vi "WritemmWavePosition.vi"(8 "error in (no error)":errorcluster, 9 "Axis Position, eng.":dbl, 10 "mmWave Axis Name":string, 11 "UI MotionStatus in":refnum<class "UI MotionStatus.lvclass">) -> (0 "error out":errorcluster, 3 "UI MotionStatus out":refnum<class "UI MotionStatus.lvclass">)   [LabVIEW 2019, in "UI MotionStatus.lvclass"]
doc: "Use mmWave axis name to find numeric indicator refnum.\nwrite value."
uses:
  UI MotionStatus.lvclass
  UI MotionStatus.lvclass/UI MotionStatus.ctl
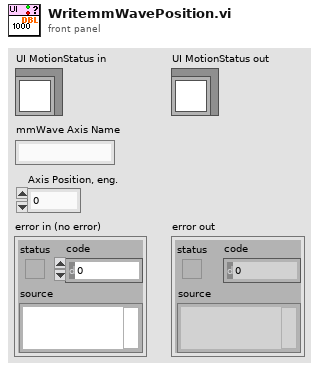
[diagram p1: front panel]
types:
  T1 = typedef "PositonIndicatorsCtrlRefs.ctl" = cluster{"BS1":refnum<vi>, "BS2":refnum<vi>, "BS3":refnum<vi>, "BS4":refnum<vi>, "RT3":refnum<vi>, "RT2":refnum<vi>, "RT1":refnum<vi>}
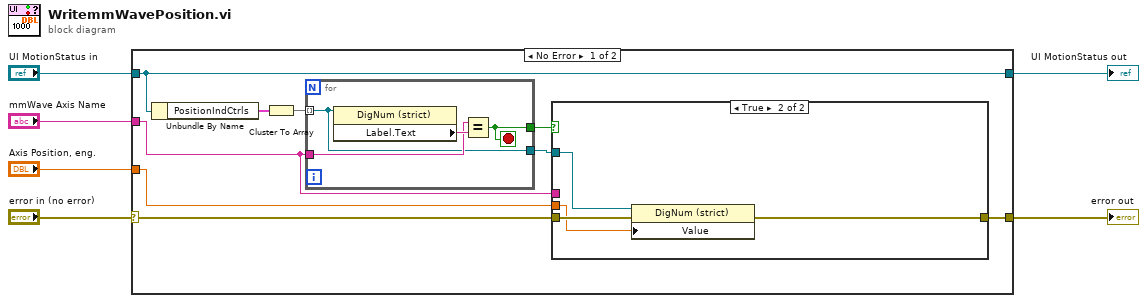
[diagram p0: block diagram]
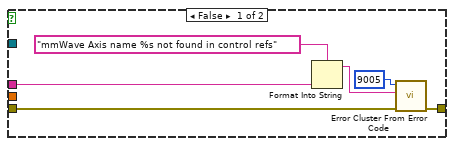
[diagram p2: hidden frame]
diagram:
  n1 = case shown="No Error" "error in (no error)" {
    selector: "error in (no error)" -> [w11 w31]
    tunnel: [w10 w31] -> w5
    tunnel: [w15 w30] -> w3
    tunnel: "UI MotionStatus in" -> [w15 w30]
    tunnel: "mmWave Axis Name" -> [w12 _]
    tunnel: "Axis Position, eng." -> [w7 _]
    frame No Error {
      n2 = Unbundle By Name(w15) -> ("PositionIndCtrls"=w14:T1)
      n3 = Cluster To Array(cluster=w14) -> (array=w13:refnum<vi>[])
      n4 = for {
        tunnel: w12 -> [w28]
        tunnel: w13 -> [w27] mode=indexing
        tunnel: [w27] -> w8
        tunnel: [w26] -> w9
        stop <- w26 stop-if-true
        n5 = property class="DigNum (strict)"(reference=w27) -> ("Label.Text"=w29:string)  [unwired: 1 in, 2 out]
        n6 = Equal?(x=w28, y=w29) -> (x = y?=w26:bool)
      }
      n7 = case shown="True" w9 {
        tunnel: w12 -> [w18 _]
        tunnel: w11 -> [w17 w24]
        tunnel: [w16 w23] -> w10
        tunnel: w8 -> [_ w25]
        tunnel: w7 -> [_ w22]
        frame False {
          n8 = Format Into String(format string="mmWave Axis name %s not found in control refs", w18) -> (resulting string=w19:string)  [unwired: 2 in, 1 out]
          n9 = call <vilib>:"Error Cluster From Error Code.vi"("error in (no error)"=w17, "error message (\"\")"=w19, "error code (0)"=9005) -> ("error out"=w16:errorcluster)  [unwired: 6 in]
        }
        frame True {
          n10 = property class="DigNum (strict)"(reference=w25, error in=w24, "Value"=w22) -> (error out=w23:errorcluster)  [unwired: 1 out]
        }
      }
    }
    frame Error {
    }
  }
  "error out" <- w5
  "UI MotionStatus out" <- w3
